vi "mks946_get_pressure.vi"(6 "err_in":errorcluster, 7 "visa_in":refnum<visa-resource-name>="COM3", 10 "channel":i32=1, 11 "address":i32=253) -> (0 "status":bool=TRUE, 2 "message":string, 3 "value":dbl, 4 "err_out":errorcluster={"status"=FALSE, "code"=1073676294, "source"="VISA Read in thcd_get_chan.vi"}, 5 "visa_out":refnum<visa-resource-name>="COM3")   [LabVIEW 2019]
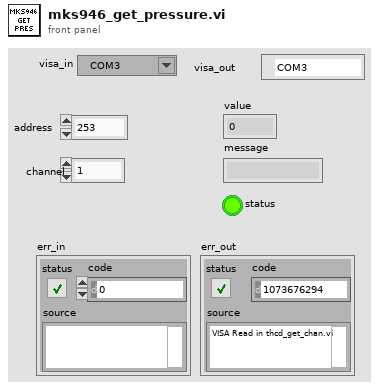
[diagram p1: front panel]
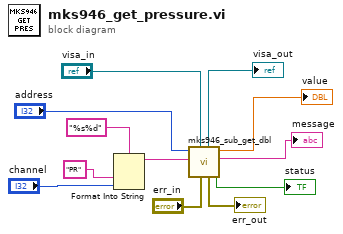
[diagram p0: block diagram]
diagram:
  n1 = Format Into String(format string="%s%d", "PR" ("mks946_comm"), "channel") -> (resulting string=w2:string)  [unwired: 2 in, 1 out]
  n2 = call "mks946_sub_get_dbl.vi"("error in (no error)"="err_in", "VISA_ref_in"="visa_in", "command"=w2, "address"="address") -> ("status"=→"status":bool, "message"=→"message":string, "value"=→"value":dbl, "error out"=→"err_out":errorcluster, "VISA_ref_out"=→"visa_out":refnum<visa-resource-name>)  [unwired: 3 in]
